vi "SRV_Build Non-Calculated Sensors Config Array.vi"(11 "Sensors Config":T1[](array[typedef]) {"Register" format="%.0x"; "I2C Address" format="%.0x"; "Sample Period (ms)" min=10 max=60000 step=1; "Digital Mask" format="%.0x"; "Channel" format="%.0x"}) -> (1 "Non-Calculated Sensors Names":string[](array[string]), 2 "Non-Calculated Sensors Config":T1[](array[typedef]) {"Register" format="%.0x"; "I2C Address" format="%.0x"; "Sample Period (ms)" min=10 max=60000 step=1; "Digital Mask" format="%.0x"; "Channel" format="%.0x"})   [LabVIEW 2009]
uses:
  SRV_Sensor Config Cluster.ctl
  SRV_Sensor Analog-Digital.ctl
  SRV_Sensor Sampling Mode.ctl
  SRV_Sensor View Config Cluster.ctl
  SRV_Sensors Names.ctl
  SRV_Sensor PicoC Shared Var Type.ctl
  SRV_Sensor Number of Bytes.ctl
  SRV_Sensor Integer Word Type.ctl
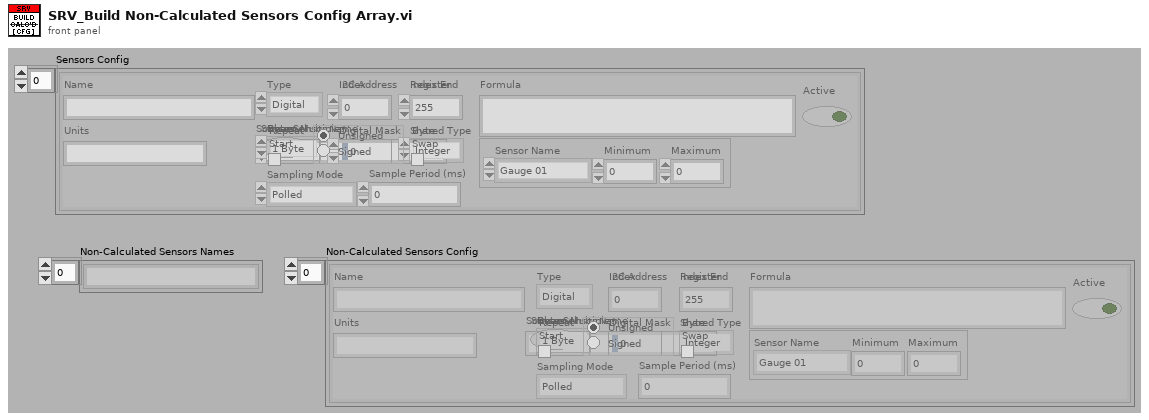
[diagram p1: front panel]
types:
  T1 = typedef "SRV_Sensor Config Cluster.ctl" = cluster{"Name":string, "A/D":T2, "I2C Address":u8, "Register":u8, "Channel":u8, "Digital Mask":u16, "Units":string, "Sampling Mode":T3, "Sample Period (ms)":u32, "Formula":string, "Sensor View Config":T4, "Active":bool, "PicoC Shared Var Type":T6, "Index":u8, "Stream Multiple?":bool, "Index End":u8, "Bytes":T7, "Source Sensor Name":string, "Repeat Start":bool, "Integer Word Type":T8, "Byte Swap":bool}
  T2 = typedef "SRV_Sensor Analog-Digital.ctl" = enum16{"Digital", "Analog", "PicoC Shared", "Calculated"}
  T3 = typedef "SRV_Sensor Sampling Mode.ctl" = enum16{"Polled", "Streaming"}
  T4 = typedef "SRV_Sensor View Config Cluster.ctl" = cluster{"Sensor Name":T5, "Minimum":dbl, "Maximum":dbl}
  T5 = typedef "SRV_Sensors Names.ctl" = enum16{"Gauge 01", "Gauge 02", "Gauge 03", "Gauge 04", "Meter 01", "Meter 02", "Meter 03", "Meter 04", "Numeric 01", "Numeric 02", "Numeric 03", "Numeric 04", "Numeric 05", "Numeric 06", "Numeric 07", "Numeric 08", "Boolean 01", "Boolean 02", "Boolean 03", "Boolean 04", "Boolean 05", "Boolean 06", "Boolean 07", "Boolean 08", "Boolean 09", "Boolean 10", "Boolean 11", "Boolean 12", "Boolean 13", "Boolean 14", "Boolean 15", "Boolean 16", "Boolean 17", "Boolean 18", "Boolean 19", "Boolean 20", "Boolean 21", "Boolean 22", "Boolean 23", "Boolean 24", "Boolean 25", "Boolean 26", "Boolean 27", "Boolean 28", "Boolean 29", "Boolean 30", "Boolean 31", "Boolean 32"}
  T6 = typedef "SRV_Sensor PicoC Shared Var Type.ctl" = enum16{"String", "Integer", "Float"}
  T7 = typedef "SRV_Sensor Number of Bytes.ctl" = enum16{"1 Byte", "2 Bytes"}
  T8 = typedef "SRV_Sensor Integer Word Type.ctl" = enum32{"Unsigned", "Signed"}
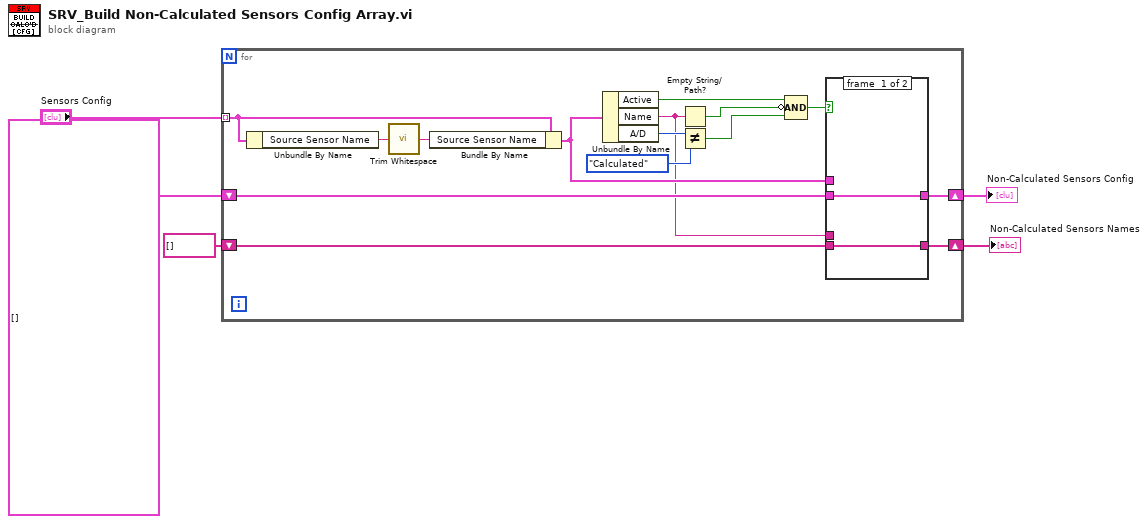
[diagram p0: block diagram]
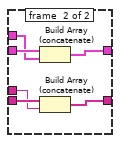
[diagram p2: hidden frame]
diagram:
  n1 = for {
    tunnel: "Sensors Config" -> [w18] mode=indexing
    shift-right: [w16] -> w3
    shift-left: T1[] [] ("Calculated Sensors Config") -> [w20]
    shift-right: [w8] -> w1
    shift-left: string[] [] -> [w7]
    n2 = Unbundle By Name(w18) -> ("Source Sensor Name"=w19:string)
    n3 = call <vilib>:"Trim Whitespace.vi"("string"=w19) -> ("trimmed string"=w17:string)  [unwired: 1 in]
    n4 = Bundle By Name(cluster=w18, "Source Sensor Name"=w17) -> (w9:T1)
    n5 = Unbundle By Name(w9) -> ("Active"=w11:bool, "Name"=w6:string, "A/D"=w13:T2)
    n6 = Empty String/Path?(string/path=w6) -> (empty?=w12:bool)
    n7 = Not Equal?(x=w13, y=SRV_Sensor_Analog-Digital."Calculated") -> (x != y?=w15:bool)
    n8 = Compound Arithmetic op=AND(w11, invert w12, w15) -> (w10:bool)
    n9 = case shown="True" w10 {
      tunnel: w20 -> [w22 w28]
      tunnel: w9 -> [_ w27]
      tunnel: [w22 w26] -> w16
      tunnel: [w21 w25] -> w8
      tunnel: w7 -> [w21 w24]
      tunnel: w6 -> [_ w23]
      frame #0 {
      }
      frame #1 {
        n10 = Build Array (concatenate)(w28, w27) -> (w26:T1[])
        n11 = Build Array (concatenate)(w24, w23) -> (w25:string[])
      }
    }
  }
  "Non-Calculated Sensors Config" <- w3
  "Non-Calculated Sensors Names" <- w1
